vi "SetTests.vi"(8 "error in (no error)":errorcluster, 10 "tests":refnum<class>[](array[class]), 11 "TestSuite in":refnum<class "TestSuite.lvclass">) -> (0 "error out":errorcluster, 3 "TestSuite in":refnum<class "TestSuite.lvclass">)   [LabVIEW 2013, in "TestSuite.lvclass"]
doc: "Sets the test members of testSuite. 'tests' can be testCase or testSuite objects (can be mixed). Note that this method should only be called after the 'Test Cases' have been created. Expected usage for this method is in TestSuite.setUp where a developer may need to call TestSuite.GetTests to get test objects and potentially modify test data and then call TestSuite.SetTests to replace the test objects. Be careful when using this method to ensure that existing Test object data used by framework is not lost or unexpected results are possible."
uses:
  TestSuite.lvclass
  TestSuite.lvclass/TestSuite.ctl
panel:
  # "JKI VI Tester for LabVIEW\nhttp://jkisoft.com/vi-tester\nCopyright (C) 2007-2009, JKI <info@jkisoft.com>\nALL RIGHTS RESERVED"
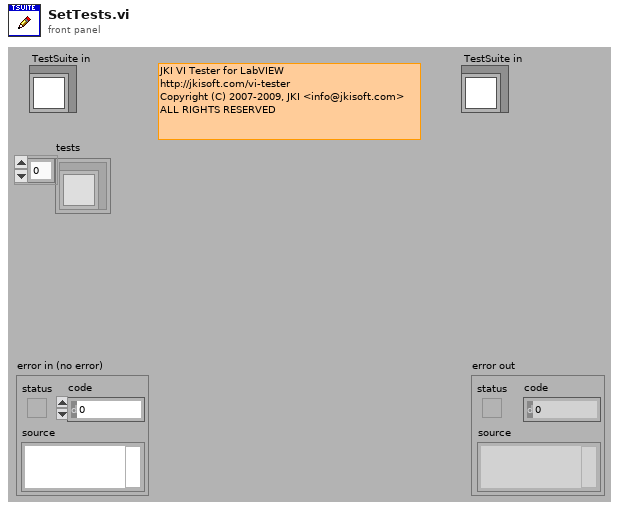
[diagram p1: front panel]
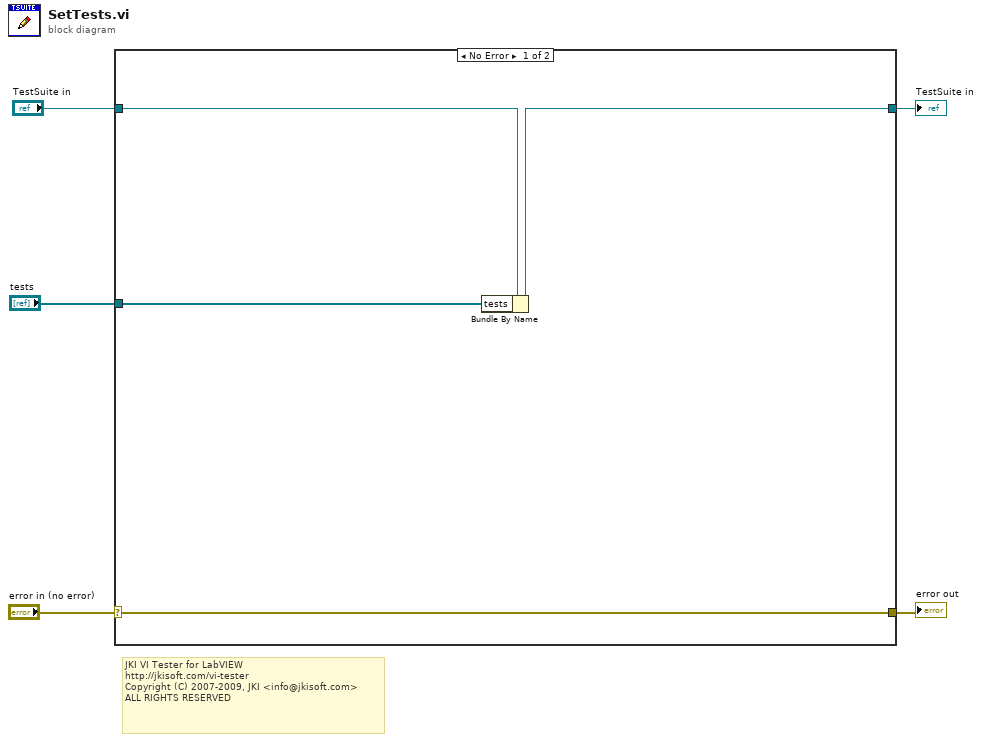
[diagram p0: block diagram]
diagram:
  # "JKI VI Tester for LabVIEW\nhttp://jkisoft.com/vi-tester\nCopyright (C) 2007-2009, JKI <info@jkisoft.com>\nALL RIGHTS RESERVED"
  n1 = case shown="No Error" "error in (no error)" {
    selector: "error in (no error)" -> [w9 w11]
    tunnel: [w9 w11] -> w4
    tunnel: [w7 w10] -> w2
    tunnel: "TestSuite in" -> [w8 w10]
    tunnel: "tests" -> [w6 _]
    frame No Error {
      n2 = Bundle By Name(cluster=w8, "tests"=w6) -> (w7:refnum<class "TestSuite.lvclass">)
    }
    frame Error {
    }
  }
  "error out" <- w4
  "TestSuite in" <- w2
